vi "Mono10 to Mono14 to U16 Array.vi"(0 "2-Byte Mono Data":u8[](array[numeric]) format="%08b", 1 "Image Size":T1) -> (2 "U16 Pixels":u16[][](array[numeric]) format="%016b")   [LabVIEW 2020, in "Buffer.lvclass"]
uses:
  Buffer.lvclass
  Image Size.ctl
  Buffer.lvclass/Buffer.ctl
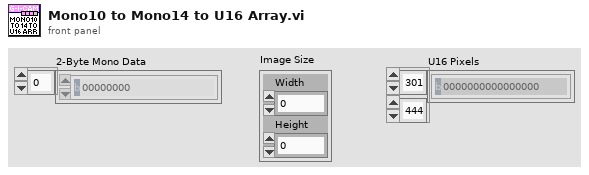
[diagram p1: front panel]
types:
  T1 = typedef "Buffer.lvclass/Image Size.ctl" = cluster{"Width":u16, "Height":u16}
  T2 = enum16{"big-endian, network order", "native, host order", "little-endian"}
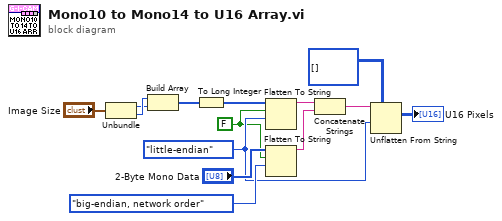
[diagram p0: block diagram]
diagram:
  w2 = T2."little-endian" ("byte order (0:big-endian, network order)")
  w1 = FALSE ("prepend array or string size? (T)")
  n1 = Unbundle("Image Size") -> ("Width"=w4:u16, "Height"=w5:u16)
  n2 = Build Array(w5, w4) -> (w3:u16[])
  n3 = To Long Integer(number=w3) -> (32bit integer=w7:i32[])
  n4 = Flatten To String(anything=w7, prepend array or string size? (T)=w1, byte order (0:big-endian, network order)=w2) -> (data string=w8:string)  [unwired: 1 in, 2 out]
  n5 = Flatten To String(anything="2-Byte Mono Data", prepend array or string size? (T)=w1, byte order (0:big-endian, network order)=T2."big-endian, network order") -> (data string=w12:string)  [unwired: 1 in, 2 out]
  n6 = Concatenate Strings(w8, w12) -> (w9:string)
  n7 = Unflatten From String(type=u16[][] [] ("unsigned 16bit integer"), binary string=w9, byte order (0:big-endian, network order)=w2) -> (value=→"U16 Pixels":u16[][])  [unwired: 2 in, 2 out]
